vi "TeleopEnqueueInput.vi"(8 "error in (no error)":errorcluster, 9 "Variant":variant, 10 "QueueEnum":T1(ring), 11 "Queue In":refnum<queue>) -> (0 "error out":errorcluster)   [LabVIEW 2012]
panel:
  out "Queue Out":refnum<queue>
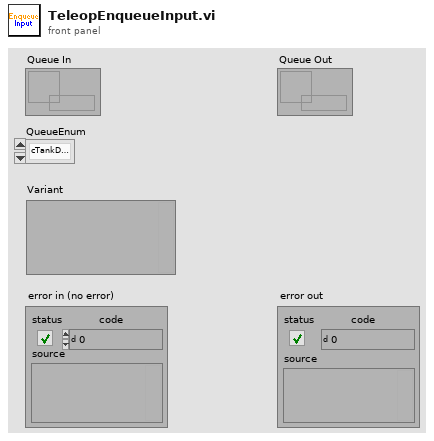
[diagram p1: front panel]
types:
  T1 = enum16{"cTankDriveLeft", "cTankDriveRight", "cHalfSpeed", "cClimbStart", "cClimbWeight", "cRpmControl", "cAngleControl", "cPresetClimbHigh", "cPresetClimbLow", "cFeederAngle", "cPresetHigh", "cLauncherAngle", "cLauncherWheel", "cFirePneumatic", "cQuickShoot", "cResetAngleEncoder"}
  T2 = cluster{"QueueEnum":enum16{"cTankDriveLeft", "cTankDriveRight", "cHalfSpeed", "cClimbStart", "cClimbWeight", "cRpmControl", "cAngleControl", "cPresetClimbHigh", "cPresetClimbLow", "cFeederAngle", "cPresetHigh", "cLauncherAngle", "cLauncherWheel", "cFirePneumatic", "cQuickShoot", "cResetAngleEncoder"}, "Variant":variant}
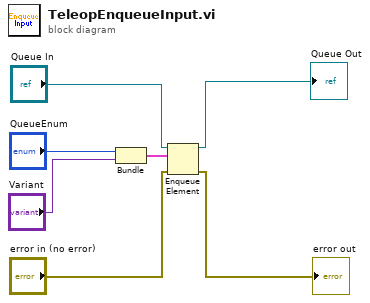
[diagram p0: block diagram]
diagram:
  n1 = Bundle("QueueEnum"="QueueEnum", "Variant"="Variant") -> (w5:T2)  [unwired: 1 in]
  n2 = Enqueue Element(queue="Queue In", element=w5, error in (no error)="error in (no error)") -> (queue out=→"Queue Out":refnum<queue>, error out=→"error out":errorcluster)  [unwired: 1 in, 1 out]
